vi "Vision Research Phantom Series PhInt PhInterpolateColor.vi"(0 "pBMIH":T3, 1 "pPixel in":u16[](array[numeric]), 2 "CFA":T1 {"CFA" items=["CFA_NONE", "CFA_VRI", "CFA_VRIV6", "CFA_BAYER", "CFA_BAYERFLIP"]}, 3 "Algorithm":T2 items=["FAST_ALGORITHM"=1, "BEST_ALGORITHM"=5, "NO_DEMOSAICING"=6], 5 "Error In (no error)":errorcluster) -> (15 "pPixel out":u16[](array[numeric]), 19 "Error Out":errorcluster)   [LabVIEW 2013, in "VRI.lvlib"]
doc: "PhInt.dll\n\nPhInterpolateColor\nvoid PhInterpolateColor(PBITMAPINFOHEADER pBMIH, PBYTE pPixel, UINT CFA, UINT Algorithm);\n\nParameter Description\npBMIH DIB header\npPixel Pixel array\nCFA Color filter array of the camera sensor. Depending on camera version it can be CFA_VRI,\n CFA_VRIV6, CFA_BAYER. This information is available from camera using the PhCon function\n GetVersion or from the SETUP structure of the cine file.\nAlgorithm Different versions of interpolation functions having different speed/quality performances\n can be selected here. Use the predefined codes BEST_ALGORITHM of FAST_ALGORITHM.\nReturn void\nComments Build a color RGB image from an uninterpolated input image that contains raw pixels from\n the sensor. The input image can be 8 or 16 bit per pixel, the result will be 24 or 48 bpp. \n The biBitCount and biSizeImage fields of the header are updated.\n The pPixel array must be allocated for the resulting color image that is three times larger\n than the original, not interpolated, array.\n When interpolating an image from a multi-head Phantom v6 camera, this function is able \n to recognize the gray heads and to interpolate only the color quarters. This is done \n using the most significant bits of the CFA selected using the TL_GRAY, TR_GRAY, \n BL_GRAY, BR_GRAY masks. The pixels from the gray heads will have their gray level\n copied three times in the result for the Blue, Green, and Red components."
uses:
  VRI.lvlib
  _Type Defs/BITMAPINFOHEADER.ctl
  _Type Defs/PhInt Algorithm.ctl
  _Type Defs/PhInt CFA.ctl
  Phantom DLLs/PhInt.dll
panel:
  # "For instructions on the use of this VI, press Ctrl+H to display the help window and move the mouse over the icon, controls, and indicators"
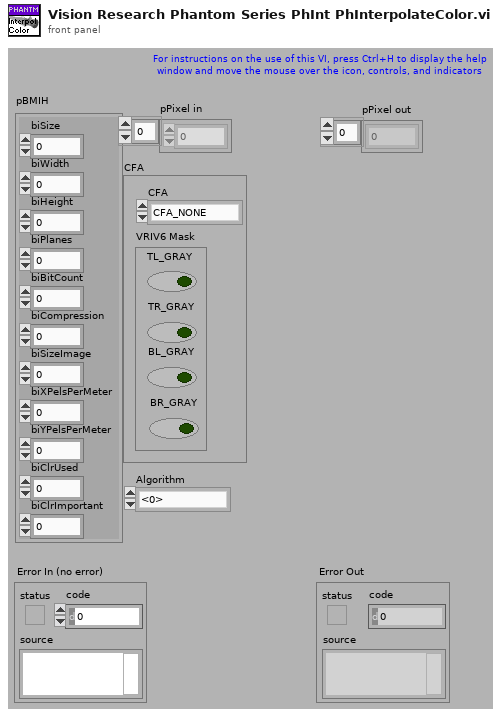
[diagram p1: front panel]
types:
  T1 = typedef "VRI.lvlib/PhInt CFA.ctl" = cluster{"CFA":u32, "VRIV6 Mask":cluster{"TL_GRAY":bool, "TR_GRAY":bool, "BL_GRAY":bool, "BR_GRAY":bool}}
  T2 = typedef "VRI.lvlib/PhInt Algorithm.ctl" = u32
  T3 = typedef "VRI.lvlib/BITMAPINFOHEADER.ctl" = cluster{"biSize":u32, "biWidth":i32, "biHeight":i32, "biPlanes":u16, "biBitCount":u16, "biCompression":u32, "biSizeImage":u32, "biXPelsPerMeter":i32, "biYPelsPerMeter":i32, "biClrUsed":u32, "biClrImportant":u32}
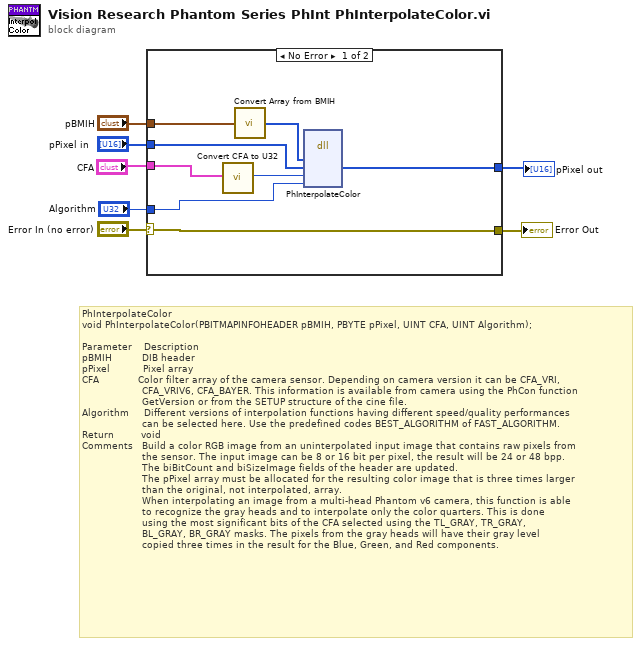
[diagram p0: block diagram]
diagram:
  # "PhInterpolateColor\nvoid PhInterpolateColor(PBITMAPINFOHEADER pBMIH, PBYTE pPixel, UINT CFA, UINT Algorithm);\n\nParameter    Description\npBMIH          DIB header\npPixel           Pixel array\nCFA             Color filter array of the camera sensor. Depending on camera version it can be CFA_VRI,\n                    CFA_VRIV6, CFA_BAYER. This information is available from camera using the PhCon function\n                    GetVersion or from the SETUP structure of the cine file.\nAlgorithm     Different versions of interpolation functions having different speed/quality performances\n                    can be selected here. Use the predefined codes BEST_ALGORITHM of FAST_ALGORITHM.\nReturn         void\nComments   Build a color RGB image from an uninterpolated input image that contains raw pixels from\n                    the sensor. The input image can be 8 or 16 bit per pixel, the result will be 24 or 48 bpp. \n                    The biBitCount and biSizeImage fields of the header are updated.\n                    The pPixel array must be allocated for the resulting color image that is three times larger\n                    than the original, not interpolated, array.\n                    When interpolating an image from a multi-head Phantom v6 camera, this function is able \n                    to recognize the gray heads and to interpolate only the color quarters. This is done \n                    using the most significant bits of the CFA selected using the TL_GRAY, TR_GRAY, \n                    BL_GRAY, BR_GRAY masks. The pixels from the gray heads will have their gray level\n                    copied three times in the result for the Blue, Green, and Red components."
  n1 = case shown="No Error" "Error In (no error)" {
    selector: "Error In (no error)" -> [w15 w16]
    tunnel: [w15 w16] -> w6
    tunnel: "pBMIH" -> [w14 _]
    tunnel: "pPixel in" -> [w13 _]
    tunnel: "CFA" -> [w12 _]
    tunnel: "Algorithm" -> [w11 _]
    tunnel: [w10 _] -> w1
    frame No Error {
      n2 = call "Convert CFA to U32.vi"("CFA in"=w12) -> ("CFA out"=w8:u32)  [unwired: 18 out]
      n3 = call "Convert Array from BMIH.vi"("BITMAPINFOHEADER"=w14) -> ("Array"=w9:u8[])
      n4 = dll-call lib="C:/Projects/SDK/32-bit/Vision Research Phantom Series Labview Driver/Phantom DLLs/PhInt.dll" fn="PhInterpolateColor"("pBMIH"=w9, "pPixel"=w13, "CFA"=w8, "Algorithm"=w11) -> ("pPixel"=w10:u16[])  [unwired: 6 in, 3 out]
    }
    frame Error {
    }
  }
  "Error Out" <- w6
  "pPixel out" <- w1
